vi "UART Read Bytes.vi"(7 "TimeOutMs":i32, 9 "pReadData":u8, 10 "Channel":u8, 11 "DevHandle":i32) -> (1 "pReadData out":u8, 3 "function return":i32)   [LabVIEW 2010, in "usb2uart.lvlib"]
doc: "int WINAPI UART_ReadBytes(int DevHandle,unsigned char Channel,unsigned char *pReadData,int TimeOutMs);"
uses:
  usb2uart.lvlib
  USB2XXX.dll
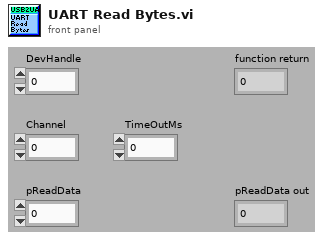
[diagram p1: front panel]
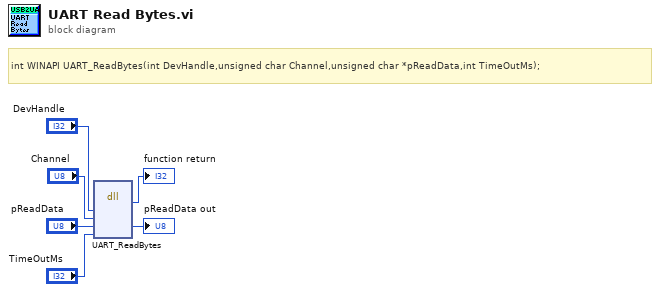
[diagram p0: block diagram]
diagram:
  # "int WINAPI UART_ReadBytes(int DevHandle,unsigned char Channel,unsigned char *pReadData,int TimeOutMs);"
  n1 = dll-call lib="E:/OtherWork/STM32/USB2XXX_Example/trunk/Labview/PublicFiles/USB2XXX.*" fn="UART_ReadBytes"("DevHandle"="DevHandle", "Channel"="Channel", "pReadData"="pReadData", "TimeOutMs"="TimeOutMs") -> (→"function return":i32, "pReadData"=→"pReadData out":u8)  [unwired: 6 in, 2 out]
